vi "SimpleSumVI.vi"(8 "Y":dbl, 9 "X":dbl) -> (3 "Result":dbl)   [LabVIEW 2023, in "SimpleClassInVi.lvclass"]
uses:
  SimpleClassInVi.lvclass
  SimpleClassInVi.lvclass/SimpleClassInVi.ctl
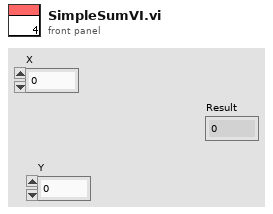
[diagram p1: front panel]
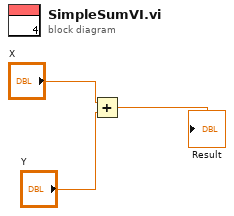
[diagram p0: block diagram]
diagram:
  n1 = Add(x="X", y="Y") -> (x+y=→"Result":dbl)
